vi "ndipolarisFileOutput-Q-vectors-TCP Server and NDI Loops - Async Comm.vi"() -> ()   [LabVIEW 2013]
panel:
  out "Stop Reading":bool
  out "Start Reading":bool
  out "Object Identifier":string
  in  "Track Outside Measurement Volume? (F:No)":bool
  in  "Track Stray Markers? (F:No)":bool
  out "Current Transformations":T1(array[cluster])
  out "NDI Readings":T2={"Port Handle"="", "Frame Number"=0, "Tx"=0.0, "Ty"=0.0, "Tz"=0.0, "Q0"=0.0, "Qx"=0.0, "Qy"=0.0, "Qz"=0.0, "Deviation"=0.0, " Markers Missing"=TRUE, "Out of Volume"=TRUE} {"Deviation" format="%#.4f"; "Qz" format="%#.4f"; "Qy" format="%#.4f"; "Qx" format="%#.4f"; "Q0" format="%#.4f"; "Tz" format="%#.2f"; "Ty" format="%#.2f"; "Tx" format="%#.2f"}
  out "TCP loop":i32
  in  "TCP Server Running":bool=TRUE
  out "Command String":string
  in  "Output Directory":path=path "C:/Users/Diogo/Desktop/NDI-Labview projects"
  out "NDI Loop":i32
  in  "NDI  Running":bool=TRUE
  in  "VISA resource name":refnum<visa-resource-name>="COM8"
  in  "Reset? (T:Yes)":bool=TRUE
  in  "Location of ROM File for Tool":path=path "C:/Program Files (x86)/Northern Digital Inc/8700248.rom"
  in  "Serial Configuration":T3={"Baud Rate (9600)"=9600, "Flow Control (0:None)"=0, "Parity"=0, "Data Bits"=8, "Stop Bits"=10} {"Stop Bits" items=["1.0"=10, "2.0"=20]; "Parity" items=["None", "Odd", "Even"]; "Flow Control (0:None)" items=["None", "XON/XOFF"]; "Baud Rate (9600)" items=["9600"=9600, "14.4k"=14400, "19.2k"=19200, "38.4k"=38400, "57.6k "=57600, "115.2k"=115200]}
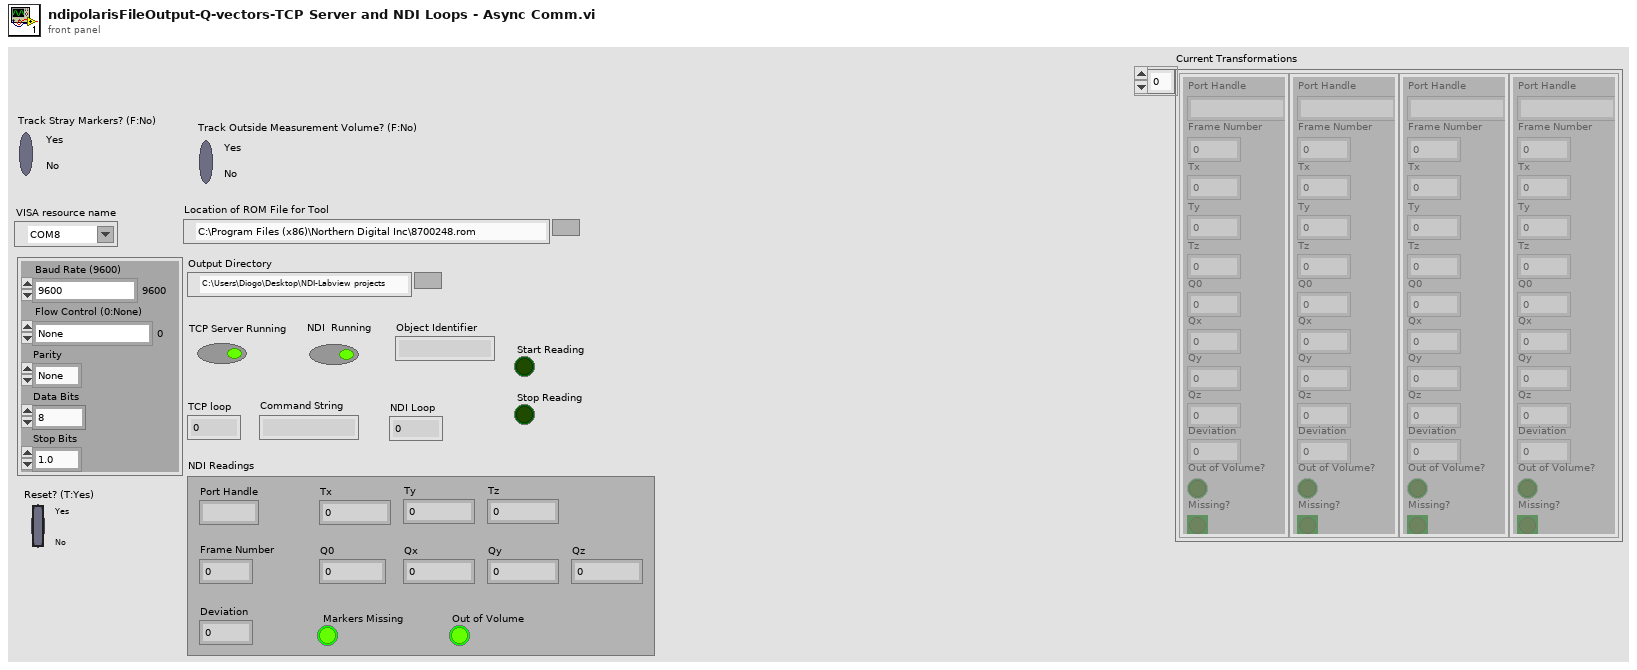
[diagram p1: front panel]
types:
  T1 = cluster{"Port Handle":string, "Frame Number":u32, "Tx":dbl, "Ty":dbl, "Tz":dbl, "Q0":dbl, "Qx":dbl, "Qy":dbl, "Qz":dbl, "Deviation":dbl, "Missing?":bool, "Out of Volume?":bool}[]
  T2 = cluster{"Port Handle":string, "Frame Number":i32, "Tx":dbl, "Ty":dbl, "Tz":dbl, "Q0":dbl, "Qx":dbl, "Qy":dbl, "Qz":dbl, "Deviation":dbl, " Markers Missing":bool, "Out of Volume":bool}
  T3 = cluster{"Baud Rate (9600)":u32, "Flow Control (0:None)":u16, "Parity":u16, "Data Bits":u16, "Stop Bits":u16}
  T4 = cluster{"Transformations[0]":cluster{"Port Handle":string, "Frame Number":u32, "Tx":dbl, "Ty":dbl, "Tz":dbl, "Q0":dbl, "Qx":dbl, "Qy":dbl, "Qz":dbl, "Deviation":dbl, "Missing?":bool, "Out of Volume?":bool}, "Transformations[1]":cluster{"Port Handle":string, "Frame Number":u32, "Tx":dbl, "Ty":dbl, "Tz":dbl, "Q0":dbl, "Qx":dbl, "Qy":dbl, "Qz":dbl, "Deviation":dbl, "Missing?":bool, "Out of Volume?":bool}, "Transformations[2]":cluster{"Port Handle":string, "Frame Number":u32, "Tx":dbl, "Ty":dbl, "Tz":dbl, "Q0":dbl, "Qx":dbl, "Qy":dbl, "Qz":dbl, "Deviation":dbl, "Missing?":bool, "Out of Volume?":bool}, "Transformations[3]":cluster{"Port Handle":string, "Frame Number":u32, "Tx":dbl, "Ty":dbl, "Tz":dbl, "Q0":dbl, "Qx":dbl, "Qy":dbl, "Qz":dbl, "Deviation":dbl, "Missing?":bool, "Out of Volume?":bool}, "Transformations[4]":cluster{"Port Handle":string, "Frame Number":u32, "Tx":dbl, "Ty":dbl, "Tz":dbl, "Q0":dbl, "Qx":dbl, "Qy":dbl, "Qz":dbl, "Deviation":dbl, "Missing?":bool, "Out of Volume?":bool}, "Transformations[5]":cluster{"Port Handle":string, "Frame Number":u32, "Tx":dbl, "Ty":dbl, "Tz":dbl, "Q0":dbl, "Qx":dbl, "Qy":dbl, "Qz":dbl, "Deviation":dbl, "Missing?":bool, "Out of Volume?":bool}, "Transformations[6]":cluster{"Port Handle":string, "Frame Number":u32, "Tx":dbl, "Ty":dbl, "Tz":dbl, "Q0":dbl, "Qx":dbl, "Qy":dbl, "Qz":dbl, "Deviation":dbl, "Missing?":bool, "Out of Volume?":bool}, "Transformations[7]":cluster{"Port Handle":string, "Frame Number":u32, "Tx":dbl, "Ty":dbl, "Tz":dbl, "Q0":dbl, "Qx":dbl, "Qy":dbl, "Qz":dbl, "Deviation":dbl, "Missing?":bool, "Out of Volume?":bool}, "Transformations[8]":cluster{"Port Handle":string, "Frame Number":u32, "Tx":dbl, "Ty":dbl, "Tz":dbl, "Q0":dbl, "Qx":dbl, "Qy":dbl, "Qz":dbl, "Deviation":dbl, "Missing?":bool, "Out of Volume?":bool}}
  T5 = cluster{"Port Handle":string, "Frame Number":u32, "Tx":dbl, "Ty":dbl, "Tz":dbl, "Q0":dbl, "Qx":dbl, "Qy":dbl, "Qz":dbl, "Deviation":dbl, "Missing?":bool, "Out of Volume?":bool}
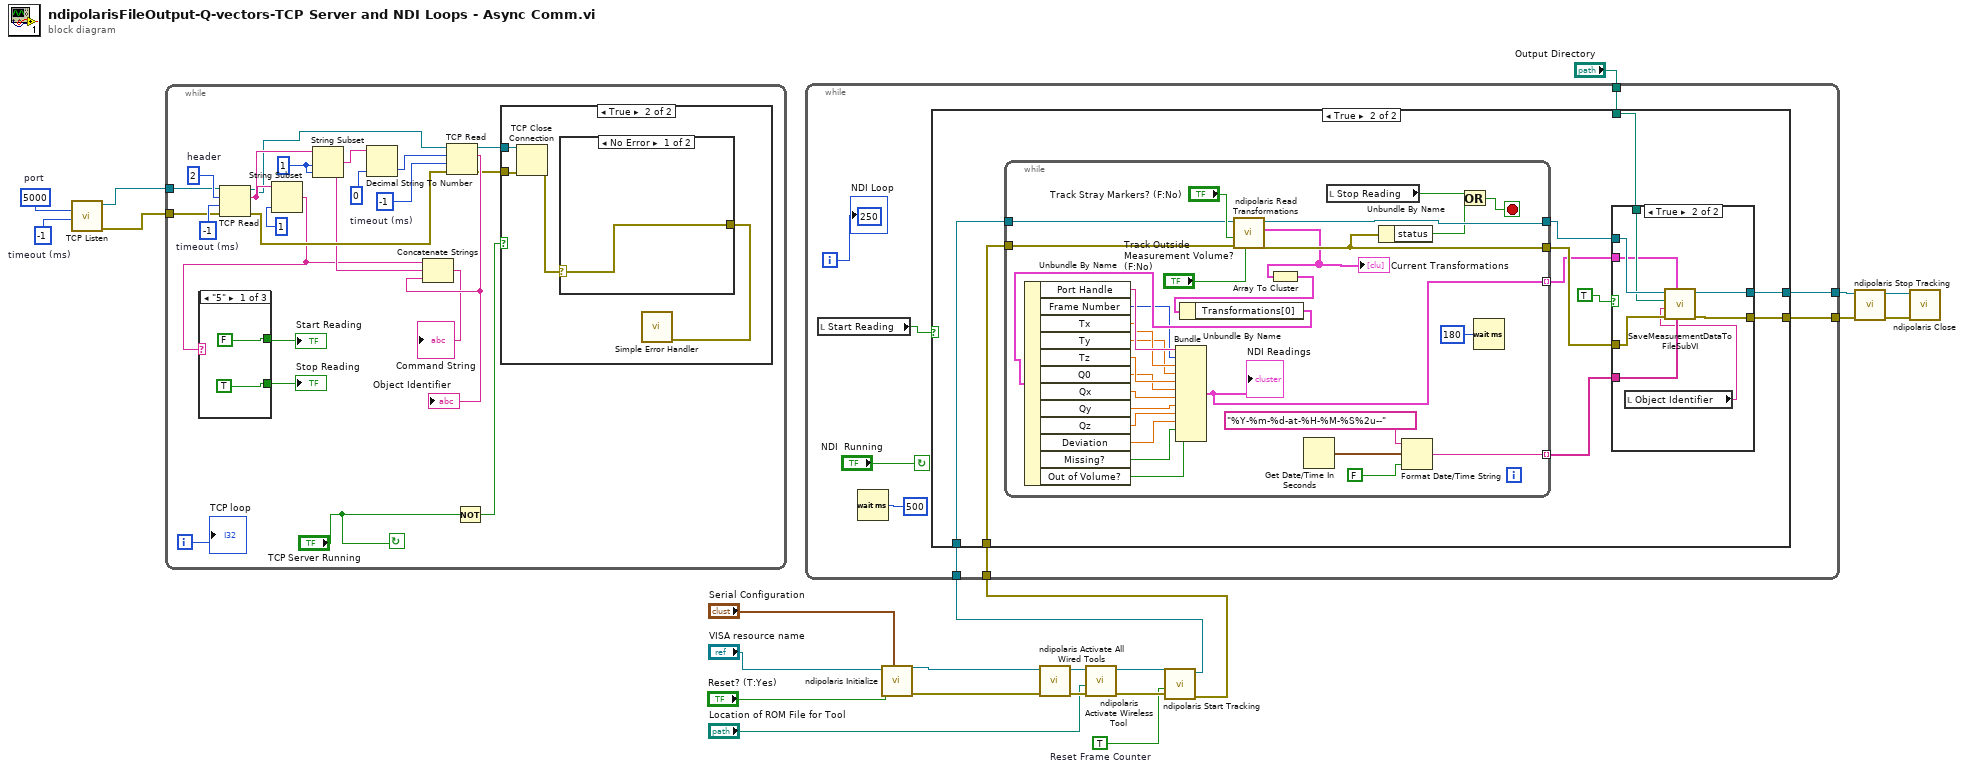
[diagram p0: block diagram]
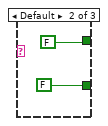
[diagram p2: hidden frame]
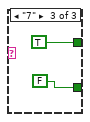
[diagram p3: hidden frame]
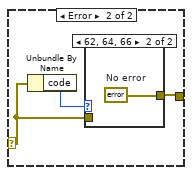
[diagram p5: hidden frame]
diagram:
  w8 = TRUE  # Reset Frame Counter
  w22 = u16 5000  # port
  w21 = i8 -1  # timeout (ms)
  n1 = call <vilib>:"TCP Listen.vi"("timeout ms (wait forever: -1)"=w21, "port"=w22) -> ("error out"=w11:errorcluster, "connection ID"=w12:refnum<k5>)  [unwired: 5 in, 3 out]
  n2 = while {
    tunnel: w12 -> [w35]
    tunnel: w11 -> [w34]
    i -> [w33]
    stop <- "TCP Server Running" continue-if-true
    w40 = u8 1 ("default (0 I32)")
    w36 = i8 -1  # timeout (ms)
    w44 = i8 -1  # timeout (ms)
    w45 = i8 2  # header
    n3 = TCP Read(connection ID=w35, bytes to read=w45, error in (no error)=w34, 9:w44) -> (connection ID out=w38:refnum<k5>, data out=w41:string, error out=w37:errorcluster)  [unwired: 1 in]
    n4 = String Subset(string=w41, length (rest)=u8 1 ("default (0 I32)")) -> (substring=w25:string)  [unwired: 1 in]
    n5 = case shown="\"5\"" w25 {
      tunnel: [FALSE FALSE TRUE] -> w24
      tunnel: [TRUE FALSE FALSE] -> w23
      frame "5" {
      }
      frame Default {
      }
      frame "7" {
      }
    }
    "Start Reading" <- w24
    "Stop Reading" <- w23
    n6 = String Subset(string=w41, offset (0)=w40, length (rest)=w40) -> (substring=w32:string)
    n7 = Decimal String To Number(string=w32, default (0L)=u8 0 ("default (0 I32)")) -> (number=w39:u8)  [unwired: 1 in, 1 out]
    n8 = TCP Read(connection ID=w38, bytes to read=w39, error in (no error)=w37, 9:w36) -> (connection ID out=w29:refnum<k5>, data out=w31:string, error out=w28:errorcluster)  [unwired: 1 in]
    "Object Identifier" <- w31
    n9 = Concatenate Strings(w25, w32, w31) -> (→"Command String":string)
    n10 = Not(x="TCP Server Running") -> (.not. x?=w27:bool)
    n11 = case shown="True" w27 {
      tunnel: w29 -> [_ w53]
      tunnel: w28 -> [_ w52]
      frame False {
      }
      frame True {
        n12 = TCP Close Connection(connection ID=w53, error in (no error)=w52) -> (error out=w54:errorcluster)  [unwired: 1 in, 1 out]
        n13 = case shown="No Error" w54 {
          selector: w54 -> [w56 w58]
          tunnel: [w56 w57] -> w55
          frame No Error {
          }
          frame Error {
            n14 = Unbundle By Name(w58) -> ("code"=w59:i32)
            n15 = case shown="62, 64, 66" w59 {
              tunnel: w58 -> [w60 _]
              tunnel: [w60 w61] -> w57
              frame Default {
              }
              frame 62, 64, 66 {
                w61 = errorcluster {"status"=FALSE, "code"=0, "source"=""}  # No error
              }
            }
          }
        }
        n16 = call <vilib>:"Simple Error Handler.vi"("error in (no error)"=w55) -> ()  [unwired: 1 in, 8 out]
      }
    }
    "TCP loop" <- w33
  }
  n17 = call <instrlib>:"ndipolaris Initialize.vi"("Serial Configuration"="Serial Configuration", "Reset? (T: Yes)"="Reset? (T:Yes)", "VISA resource name"="VISA resource name") -> ("error out"=w17:errorcluster, "VISA resource name out"=w18:refnum<visa-resource-name>)  [unwired: 7 in]
  n18 = call <instrlib>:"ndipolaris Activate All Wired Tools.vi"("error in (no error)"=w17, "VISA resource name"=w18) -> ("error out"=w19:errorcluster, "VISA resource out"=w20:refnum<visa-resource-name>)  [unwired: 7 in, 1 out]
  n19 = call <instrlib>:"ndipolaris Activate Wireless Tool.vi"("error in (no error)"=w19, "Location of ROM File for Tool"="Location of ROM File for Tool", "VISA resource name"=w20) -> ("error out"=w9:errorcluster, "VISA resource out"=w10:refnum<visa-resource-name>)  [unwired: 6 in, 1 out]
  n20 = call <instrlib>:"ndipolaris Start Tracking.vi"("error in (no error)"=w9, "Reset Frame Counter? (F:No)"=w8, "VISA resource name"=w10) -> ("error out"=w3:errorcluster, "VISA resource out"=w7:refnum<visa-resource-name>)  [unwired: 7 in]
  n21 = while {
    tunnel: w7 -> [w69]
    tunnel: [w68] -> w4
    tunnel: w3 -> [w66]
    tunnel: "Output Directory" -> [w65]
    tunnel: [w64] -> w1
    i -> [w70]
    stop <- "NDI  Running" continue-if-true
    (unwired) u8 250
    n22 = local read "Start Reading"() -> (w62:bool)
    n23 = Wait (ms)(milliseconds to wait=u32 500) -> ()  [unwired: 1 out]
    n24 = case shown="True" w62 {
      tunnel: w69 -> [w72 w82]
      tunnel: [w72 w78] -> w68
      tunnel: w66 -> [w71 w81]
      tunnel: w65 -> [_ w80]
      tunnel: [w71 w77] -> w64
      frame False {
      }
      frame True {
        n25 = while {
          tunnel: [w121] -> w74
          tunnel: [w120] -> w79
          tunnel: [w96] -> w75 mode=indexing
          tunnel: [w98] -> w76 mode=indexing
          tunnel: w82 -> [w95]
          tunnel: w81 -> [w94]
          stop <- w122 stop-if-true
          n26 = call <instrlib>:"ndipolaris Read Transformations.vi"("Track Outside Measurement Volume? (F:No)"="Track Outside Measurement Volume? (F:No)", "error in (no error)"=w94, "Track Stray Markers? (F:No)"="Track Stray Markers? (F:No)", "VISA resource name"=w95) -> ("error out"=w120:errorcluster, "Transformations"=w105:T1, "VISA resource out"=w121:refnum<visa-resource-name>)  [unwired: 4 in, 1 out]
          "Current Transformations" <- w105
          n27 = Array To Cluster(array=w105) -> (cluster=w116:T4)
          n28 = Unbundle By Name(w116) -> ("Transformations[0]"=w115:T5)
          n29 = Unbundle By Name(w115) -> ("Port Handle"=w114:string, "Frame Number"=w113:u32, "Tx"=w112:dbl, "Ty"=w111:dbl, "Tz"=w110:dbl, "Q0"=w109:dbl, "Qx"=w108:dbl, "Qy"=w107:dbl, "Qz"=w106:dbl, "Deviation"=w104:dbl, "Missing?"=w103:bool, "Out of Volume?"=w102:bool)
          n30 = Bundle("Port Handle"=w114, "Frame Number"=w113, "Tx"=w112, "Ty"=w111, "Tz"=w110, "Q0"=w109, "Qx"=w108, "Qy"=w107, "Qz"=w106, "Deviation"=w104, "Missing?"=w103, "Out of Volume?"=w102) -> (w96:T5)  [unwired: 1 in]
          "NDI Readings" <- w96
          n31 = Get Date/Time In Seconds() -> (seconds since 1Jan1904=w101:timestamp)
          n32 = local read "Stop Reading"() -> (w93:bool)
          n33 = Unbundle By Name(w120) -> ("status"=w119:bool)
          n34 = Format Date/Time String(time format string (%c)="%Y-%m-%d-at-%H-%M-%S%2u--", seconds (now)=w101, UTC format=FALSE) -> (date/time string=w98:string)
          n35 = Or(x=w93, y=w119) -> (x .or. y?=w122:bool)
          n36 = Wait (ms)(milliseconds to wait=u32 180) -> ()  [unwired: 1 out]
        }
        n37 = case shown="True" TRUE {
          tunnel: w80 -> [_ w91]
          tunnel: w79 -> [w83 w90]
          tunnel: [w84 w87] -> w78
          tunnel: [w83 w86] -> w77
          tunnel: w76 -> [_ w88]
          tunnel: w75 -> [_ w89]
          tunnel: w74 -> [w84 w92]
          frame False {
          }
          frame True {
            n38 = local read "Object Identifier"() -> (w85:string)
            n39 = call "SaveMeasurementDataToFileSubVI.vi"("Array of Time for Measurement"=w88, "Array of Measurement"=w89, "error in (no error)"=w90, "Object number"=w85, "Output Directory"=w91, "VISA Refnum in"=w92) -> ("error out"=w86:errorcluster, "VISA Refnum out"=w87:refnum<visa-resource-name>)  [unwired: 4 in]
          }
        }
      }
    }
    "NDI Loop" <- w70
  }
  n40 = call <instrlib>:"ndipolaris Stop Tracking.vi"("error in (no error)"=w1, "VISA resource name"=w4) -> ("error out"=w5:errorcluster, "VISA resource out"=w6:refnum<visa-resource-name>)  [unwired: 8 in]
  n41 = call <instrlib>:"ndipolaris Close.vi"("error in (no error)"=w5, "VISA resource name"=w6) -> ()  [unwired: 9 in, 1 out]
